vi "x502_set_cycle_signal.vi"(2 "Autostart":bool=TRUE, 3 "DAC Signals":dbl[][](array[numeric]), 4 "error in (no error)":errorcluster, 5 "x502 in":refnum<k24>) -> (0 "error out":errorcluster, 1 "x502 out":refnum<k24>)   [LabVIEW 2010]
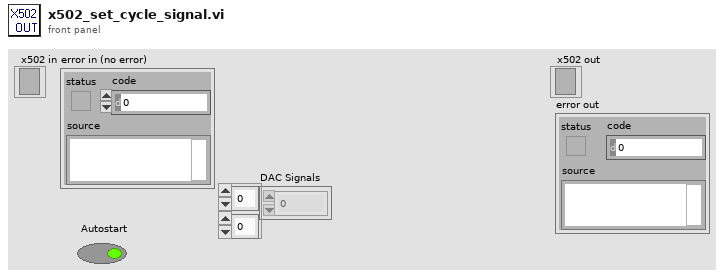
[diagram p1: front panel]
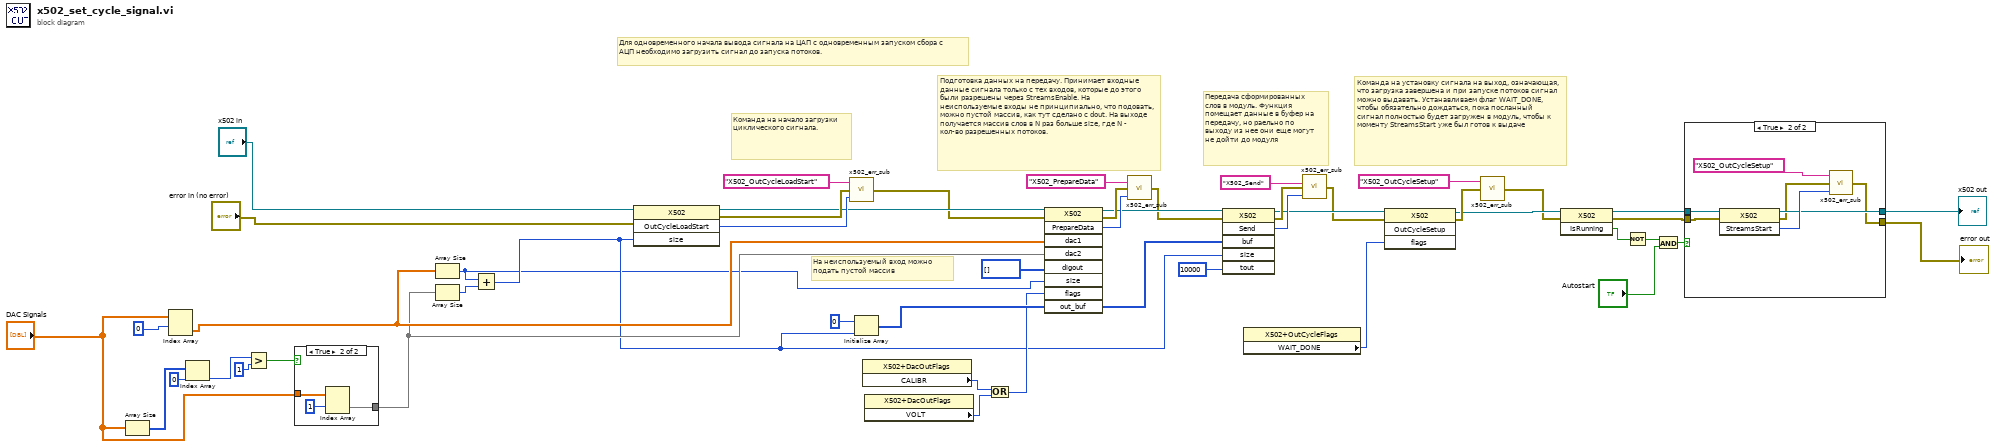
[diagram p0: block diagram]
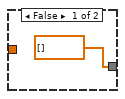
[diagram p3: hidden frame]
diagram:
  # "Команда на установку сигнала на выход, означающая, что загрузка завершена и при запуске потоков сигнал можно выдавать. Устанавливаем флаг WAIT_DONE, чтобы обязательно дождаться, пока посланный сигнал полностью будет загружен в модуль, чтобы к моменту StreamsStart уже был готов к выдаче"
  # "Передача сформированных слов в модуль. Функция помещает данные в буфер на передачу, но раельно по выходу из нее они еще могут не дойти до модуля"
  # "Подготовка данных на передачу. Принимает входные данные сигнала только с тех входов, которые до этого были разрешены через StreamsEnable. На неиспользуемые входы не принципиально, что подовать, можно пустой массив, как тут сделано с dout. На выходе получается массив слов в N раз больше size, где N - кол-во разрешенных потоков."
  # "Команда на начало загрузки циклического сигнала."
  # "Для одновременного начала вывода сигнала на ЦАП с одновременным запуском сбора с АЦП необходимо загрузить сигнал до запуска потоков."
  # "На неиспользуемый вход можно подать пустой массив"
  n1 = Array Size(array="DAC Signals") -> (size(s)=w21:i32[])
  n2 = Index Array(array="DAC Signals", index (row)=u32 0 ("element")) -> (element=w19:dbl[])  [unwired: 1 in]
  n3 = Index Array(array=w21, index=u32 0 ("element")) -> (element=w22:i32)
  n4 = Greater?(x=w22, y=u32 1 ("element")) -> (0:w23:bool)
  n5 = case shown="True" w23 {
    tunnel: "DAC Signals" -> [_ w54]
    tunnel: [dbl[] [] w52] -> w18
    frame False {
    }
    frame True {
      n6 = Index Array(array=w54, index (row)=u32 1 ("element")) -> (element=w52:dbl[])  [unwired: 1 in]
    }
  }
  n7 = Array Size(array=w19) -> (size(s)=w1:i32)
  n8 = Array Size(array=w18) -> (size(s)=w17:i32)
  n9 = Add(x=w1, y=w17) -> (x+y=w2:i32)
  n10 = invoke class="X502" method="OutCycleLoadStart"(reference="x502 in", error in="error in (no error)", "size"=w2) -> (reference out=w47:refnum<k24>, error out=w49:errorcluster, "OutCycleLoadStart"=w50:i32)  [unwired: 1 in, 1 out]
  n11 = call "x502_err_sub.vi"("Error code"=w50, "error in (no error)"=w49, "Error descr"="X502_OutCycleLoadStart") -> ("error out"=w46:errorcluster)
  n12 = Initialize Array(u32 0 ("element"), w2) -> (w43:u32[])
  n13 = property class="X502+DacOutFlags"() -> ("CALIBR"=w16:u32)  [unwired: 2 in, 2 out]
  n14 = property class="X502+DacOutFlags"() -> ("VOLT"=w15:u32)  [unwired: 2 in, 2 out]
  n15 = Or(x=w16, y=w15) -> (x .or. y?=w14:u32)
  n16 = invoke class="X502" method="PrepareData"(reference=w47, error in=w46, "dac1"=w19, "dac2"=w18, "digout"=i32[] [], "size"=w1, "flags"=w14, "out_buf"=w43) -> (reference out=w39:refnum<k24>, error out=w40:errorcluster, "PrepareData"=w41:i32, "out_buf"=w38:u32[])  [unwired: 1 in, 5 out]
  n17 = call "x502_err_sub.vi"("Error code"=w41, "error in (no error)"=w40, "Error descr"="X502_PrepareData") -> ("error out"=w36:errorcluster)
  n18 = invoke class="X502" method="Send"(reference=w39, error in=w36, "buf"=w38, "size"=w2, "tout"=u32 10000 ("element")) -> (reference out=w32:refnum<k24>, error out=w33:errorcluster, "Send"=w34:i32)  [unwired: 1 in, 3 out]
  n19 = property class="X502+OutCycleFlags"() -> ("WAIT_DONE"=w28:u32)  [unwired: 2 in, 2 out]
  n20 = call "x502_err_sub.vi"("Error code"=w34, "error in (no error)"=w33, "Error descr"="X502_Send") -> ("error out"=w31:errorcluster)
  n21 = invoke class="X502" method="OutCycleSetup"(reference=w32, error in=w31, "flags"=w28) -> (reference out=w12:refnum<k24>, error out=w29:errorcluster)  [unwired: 1 in, 2 out]
  n22 = call "x502_err_sub.vi"("error in (no error)"=w29, "Error descr"="X502_OutCycleSetup") -> ("error out"=w11:errorcluster)  [unwired: 1 in]
  n23 = invoke class="X502" method="IsRunning"(reference=w12, error in=w11) -> (reference out=w10:refnum<k24>, error out=w9:errorcluster, "IsRunning"=w4:bool)  [unwired: 1 in]
  n24 = Not(x=w4) -> (.not. x?=w5:bool)
  n25 = And(x=w5, y="Autostart") -> (x .and. y?=w6:bool)
  n26 = case shown="True" w6 {
    tunnel: w10 -> [w56 w63]
    tunnel: w9 -> [w55 w61]
    tunnel: [w56 w59] -> w8
    tunnel: [w55 w57] -> w7
    frame False {
    }
    frame True {
      n27 = invoke class="X502" method="StreamsStart"(reference=w63, error in=w61) -> (reference out=w59:refnum<k24>, error out=w58:errorcluster, "StreamsStart"=w60:i32)  [unwired: 1 in]
      n28 = call "x502_err_sub.vi"("Error code"=w60, "error in (no error)"=w58, "Error descr"="X502_OutCycleSetup") -> ("error out"=w57:errorcluster)
    }
  }
  "x502 out" <- w8
  "error out" <- w7
